vi "Untitled 1.vi"() -> ()   [LabVIEW 2015]
panel:
  out "Numeric 7":dbl
  out "Numeric 6":dbl
  out "Numeric 5":dbl
  out "Numeric 4":dbl
  out "Numeric 3":dbl
  out "Numeric 2":dbl
  out "aritmetik ortalama":dbl
  out "toplam":dbl
  out "eleman sayısı":dbl
  in  "Array":dbl[](array[numeric])
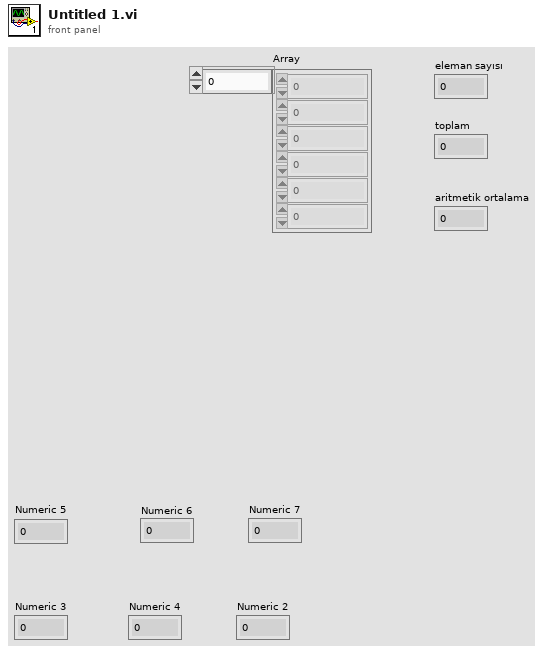
[diagram p1: front panel]
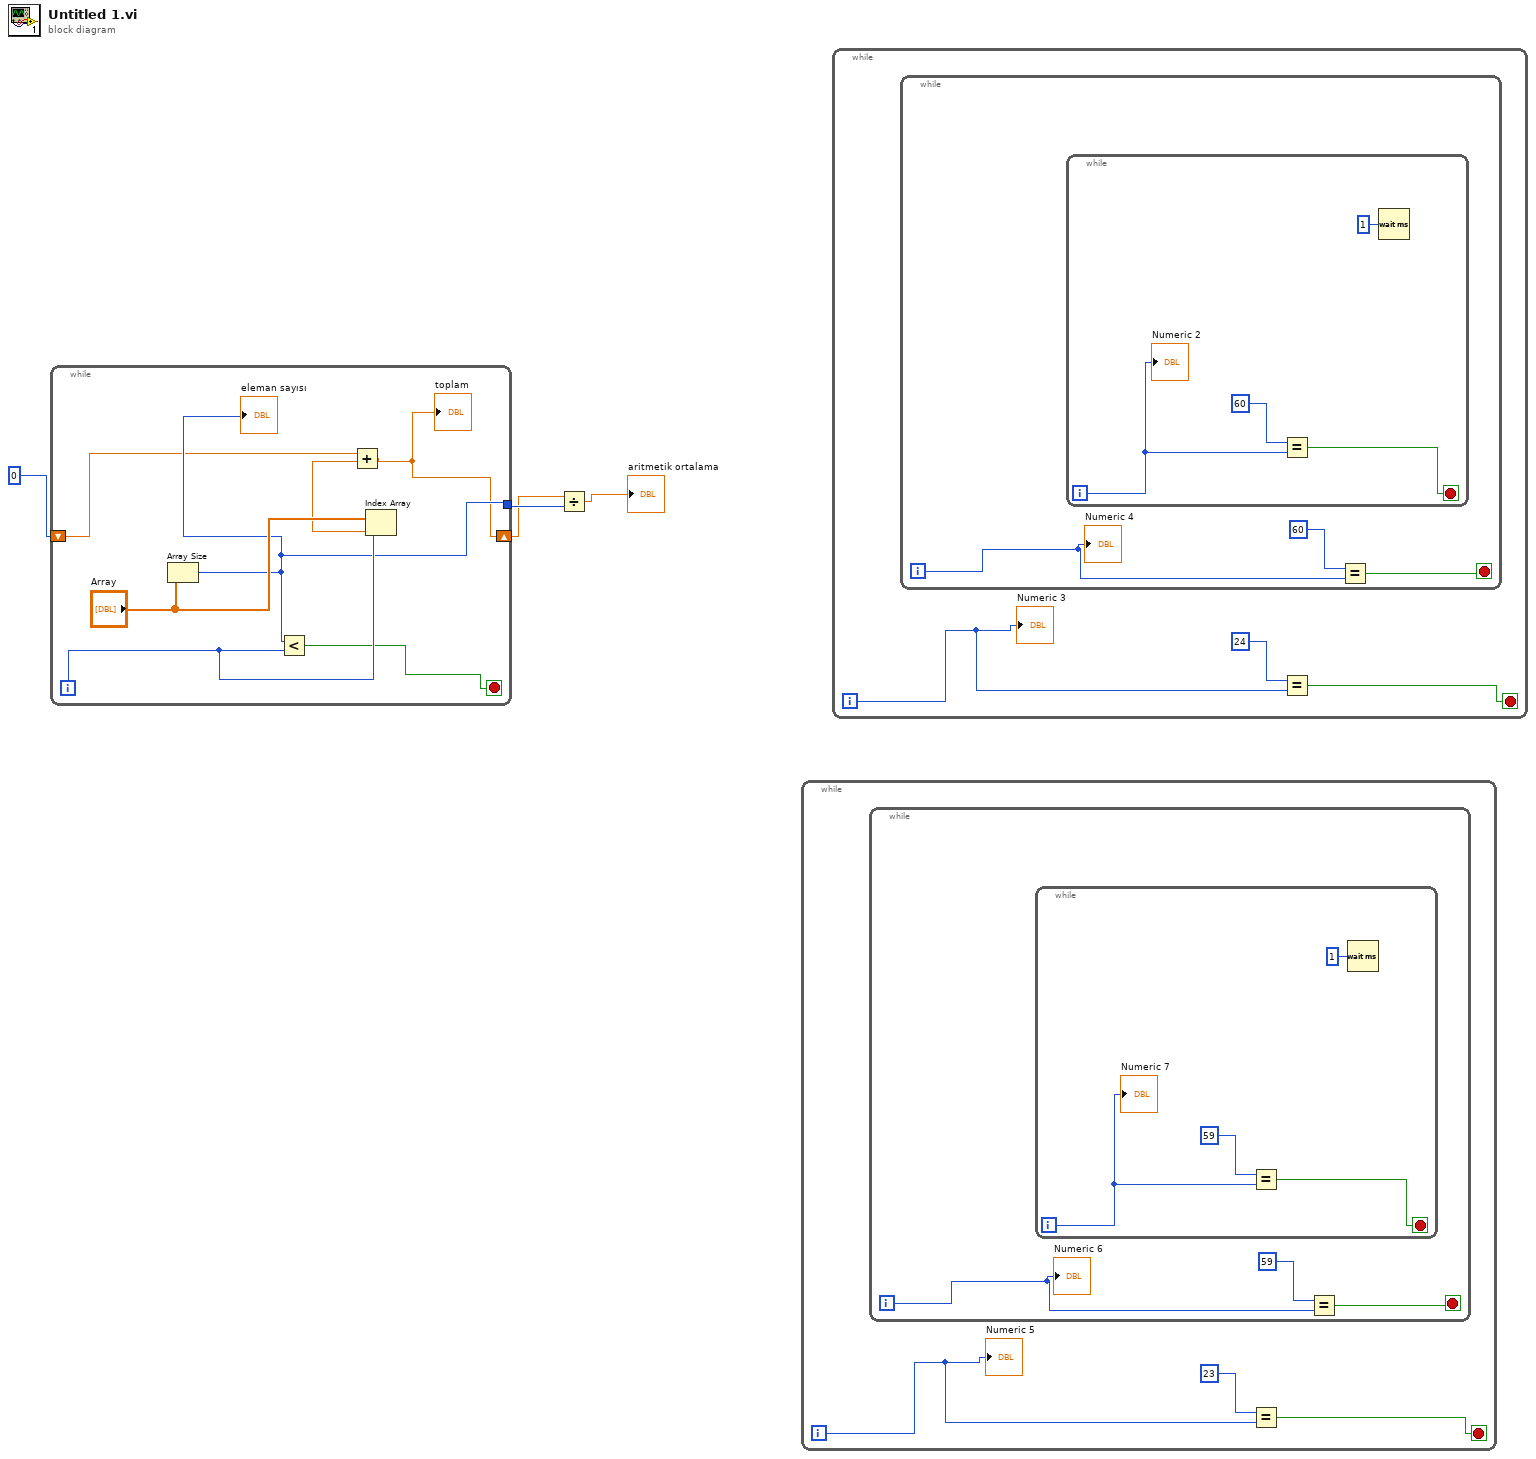
[diagram p0: block diagram]
diagram:
  n1 = while {
    shift-right: [w6] -> w2
    shift-left: 0 -> [w5]
    tunnel: [w8] -> w4
    i -> [w10]
    stop <- w9 stop-if-true
    n2 = Array Size(array="Array") -> (size(s)=w8:i32)
    "eleman sayısı" <- w8
    n3 = Less?(x=w8, y=w10) -> (x < y?=w9:bool)
    n4 = Index Array(array="Array", index=w10) -> (element=w7:dbl)
    n5 = Add(x=w5, y=w7) -> (x+y=w6:dbl)
    "toplam" <- w6
  }
  n6 = Divide(x=w2, y=w4) -> (x/y=→"aritmetik ortalama":dbl)
  n7 = while {
    i -> [w12]
    stop <- w13 stop-if-true
    n8 = while {
      i -> [w15]
      stop <- w16 stop-if-true
      n9 = while {
        i -> [w20]
        stop <- w19 stop-if-true
        n10 = Equal?(x=59, y=w20) -> (x = y?=w19:bool)
        n11 = Wait (ms)(milliseconds to wait=u32 1) -> ()  [unwired: 1 out]
        "Numeric 7" <- w20
      }
      n12 = Equal?(x=59, y=w15) -> (x = y?=w16:bool)
      "Numeric 6" <- w15
    }
    n13 = Equal?(x=23, y=w12) -> (x = y?=w13:bool)
    "Numeric 5" <- w12
  }
  n14 = while {
    i -> [w22]
    stop <- w23 stop-if-true
    n15 = while {
      i -> [w25]
      stop <- w26 stop-if-true
      n16 = while {
        i -> [w30]
        stop <- w29 stop-if-true
        n17 = Equal?(x=60, y=w30) -> (x = y?=w29:bool)
        n18 = Wait (ms)(milliseconds to wait=u32 1) -> ()  [unwired: 1 out]
        "Numeric 2" <- w30
      }
      n19 = Equal?(x=60, y=w25) -> (x = y?=w26:bool)
      "Numeric 4" <- w25
    }
    n20 = Equal?(x=24, y=w22) -> (x = y?=w23:bool)
    "Numeric 3" <- w22
  }
